vi "localArquivo.vi"(9 "extensão":string, 10 "Nome do arquivo":string, 11 "Local":path) -> (3 "Path":path)   [LabVIEW 2012]
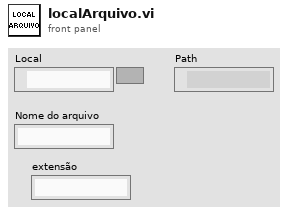
[diagram p1: front panel]
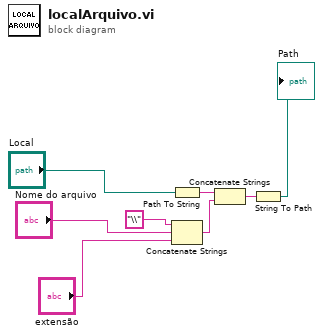
[diagram p0: block diagram]
diagram:
  n1 = Path To String(path="Local") -> (string=w3:string)
  n2 = Concatenate Strings("\\", "Nome do arquivo", "extensão") -> (w2:string)
  n3 = Concatenate Strings(w3, w2) -> (w4:string)
  n4 = String To Path(string=w4) -> (path=→"Path":path)
